vi "Start.vi"(8 "error in (no error)":errorcluster, 11 "Stream in":refnum<class "Stream.lvclass">) -> (0 "error out":errorcluster, 3 "Stream":refnum<class "Stream.lvclass">)   [LabVIEW 2020, in "capture.lvlib" / "Stream.lvclass"]
doc: "Start the Stream. This will trigger the capture device to begin capturing data which can be copied into an Image using Next Capture.vi."
uses:
  Stream.lvclass
  Stream.lvclass/Stream.ctl
  common/common.lvlib
  common/bin/gartoolkit_32-1.dll
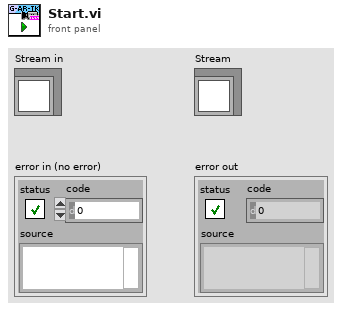
[diagram p1: front panel]
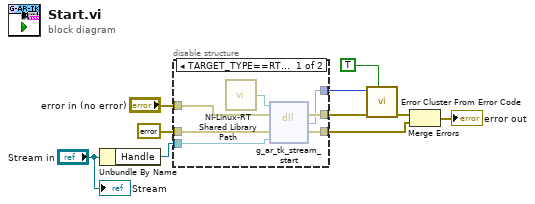
[diagram p0: block diagram]
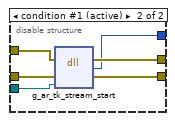
[diagram p2: hidden frame]
diagram:
  n1 = Unbundle By Name("Stream in") -> ("Handle"=w5:refnum<data-value>)
  n2 = disable-structure shown="TARGET_TYPE==RT&&OS==Linux" {
    disable-tunnel: "error in (no error)" -> [w17 w23]
    disable-tunnel: errorcluster {"status"=FALSE, "code"=0, "source"=""} ("error constant") -> [w16 w22]
    disable-tunnel: w5 -> [w15 w21]
    disable-tunnel: [w14 w20] -> w4
    disable-tunnel: [w13 w19] -> w3
    disable-tunnel: [w12 w18] -> w2
    frame condition #0 {
      n3 = call "NI-Linux-RT Shared Library Path.vi"() -> ("Path"=w11:path)
      n4 = dll-call lib="?" fn="g_ar_tk_stream_start"(path in=w11, error in=w17, "error_cluster"=w16, "EDVR_strm"=w15) -> (error out=w14:errorcluster, "MgErr"=w13:i32, "error_cluster"=w12:errorcluster)  [unwired: 2 in, 1 out]
    }
    frame condition #1 (active) {
      n5 = dll-call lib="C:/serenial/lib/g-augmented-reality-toolkit/LabVIEW/common/bin/gartoolkit_*-1.*" fn="g_ar_tk_stream_start"(error in=w23, "error_cluster"=w22, "EDVR_strm"=w21) -> (error out=w20:errorcluster, "MgErr"=w19:i32, "error_cluster"=w18:errorcluster)  [unwired: 3 in, 1 out]
    }
  }
  n6 = call <vilib>:"Error Cluster From Error Code.vi"("show call chain? (False)"=TRUE, "error in (no error)"=w4, "error code (0)"=w3) -> ("error out"=w8:errorcluster)  [unwired: 6 in]
  n7 = Merge Errors(w8, w2) -> (→"error out":errorcluster)
  "Stream" <- "Stream in"
